vi "Inside.vi"(10 "Current_char":string, 11 "Accumulator":refnum<class "Accumulator.lvclass">) -> (2 "Inside?":bool, 3 "Accumulator'":refnum<class "Accumulator.lvclass">)   [LabVIEW 2020, in "Accumulator.lvclass"]
uses:
  Accumulator.lvclass
  Accumulator.lvclass/Accumulator.ctl
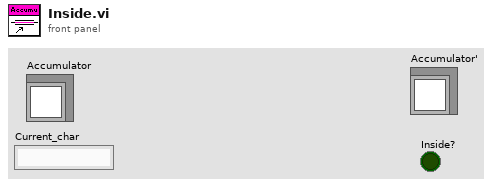
[diagram p1: front panel]
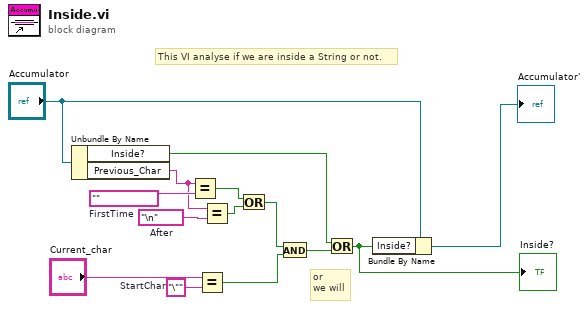
[diagram p0: block diagram]
diagram:
  w10 = "\n"  # After
  w11 = ""  # FirstTime
  w13 = "\""  # StartChar
  # "or\nwe will"
  # "This VI analyse if we are inside a String or not."
  n1 = Unbundle By Name("Accumulator") -> ("Inside?"=w3:bool, "Previous_Char"=w9:string)
  n2 = Equal?(x=w9, y=w11) -> (x = y?=w8:bool)
  n3 = Equal?(x="Current_char", y=w13) -> (x = y?=w5:bool)
  n4 = Equal?(x=w9, y=w10) -> (x = y?=w7:bool)
  n5 = Or(x=w8, y=w7) -> (x .or. y?=w6:bool)
  n6 = And(x=w6, y=w5) -> (x .and. y?=w2:bool)
  n7 = Or(x=w3, y=w2) -> (x .or. y?=w1:bool)
  "Inside?" <- w1
  n8 = Bundle By Name(cluster="Accumulator", "Inside?"=w1) -> (→"Accumulator'":refnum<class "Accumulator.lvclass">)
